vi "Read Arena Config File.vi"(8 "error in (no error)":errorcluster, 11 "Config index":i32) -> (0 "error out":errorcluster, 3 "Panel -> Bus":u8[](array[numeric]))   [LabVIEW 2013]
doc: "Reads the arena config file and extracts the Bus # of each panel. Index+1 is the Panel number."
uses:
  HHMI - Filepaths global.vi
panel:
  out "data":u8[](array[numeric])
  in  "byte order":T1(ring)
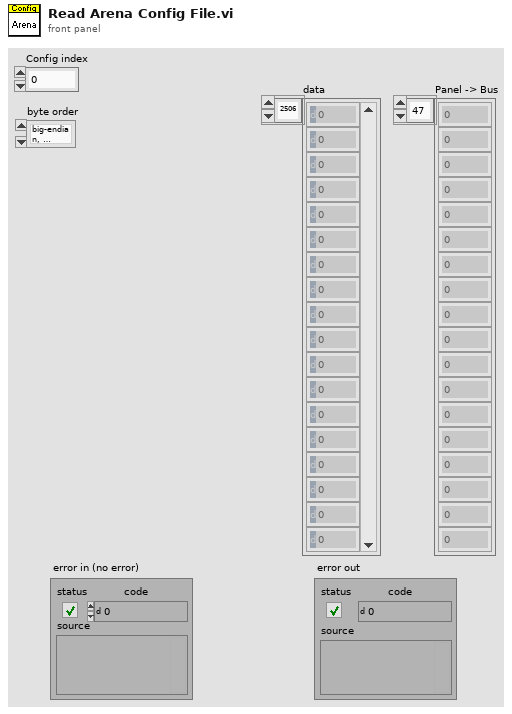
[diagram p1: front panel]
types:
  T1 = enum16{"big-endian, network order", "native, host order", "little-endian"}
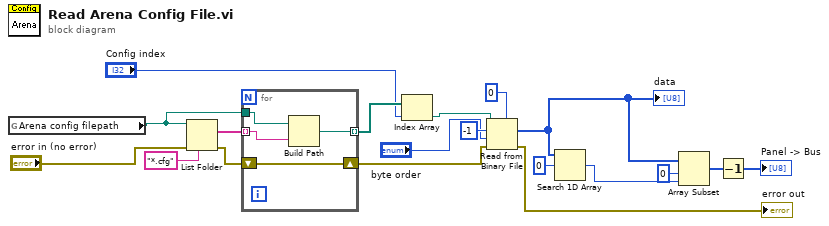
[diagram p0: block diagram]
diagram:
  n1 = global read "HHMI - Filepaths global.vi" "Arena config filepath"() -> (w1:path)
  n2 = List Folder(path=w1, pattern="*.cfg", error in="error in (no error)") -> (filenames=w9:string[], error out=w8:errorcluster)  [unwired: 1 in, 2 out]
  n3 = for {
    tunnel: w9 -> [w22] mode=indexing
    tunnel: w1 -> [w23]
    tunnel: [w21] -> w5 mode=indexing
    shift-right: [w20] -> w2
    shift-left: w8 -> [w20]
    n4 = Build Path(base path=w23, name or relative path=w22) -> (appended path=w21:path)
  }
  n5 = Index Array(array=w5, index="Config index") -> (element=w3:path)
  n6 = Read from Binary File(5:u8 0, 8:w2, 9:"byte order", 10:-1 ("count (1)"), 11:w3) -> (0:→"error out":errorcluster, 2:w16:u8[])  [unwired: 1 in, 2 out]
  "data" <- w16
  n7 = Search 1D Array(1D array=w16, element=u8 0) -> (index of element=w15:i32)  [unwired: 1 in]
  n8 = Array Subset(array=w16, index=0, length=w15) -> (w13:u8[])
  n9 = Decrement(x=w13) -> (x-1=→"Panel -> Bus":u8[])
